vi "PID Robot Drive.vi"(8 "dt":dbl, 9 "Right RPS":dbl(slide) scale=-14.75..14.75, 10 "Left RPS":dbl(slide) scale=-14.75..14.75, 11 "Robot Mode Call Context":T1) -> (0 "Right Throttle":dbl, 3 "Left Throttle":dbl)   [LabVIEW 2016]
uses:
  <vilib>/Rock Robotics/WPI/DriverStation/WPI_DriverStationDerivedRobotMode.ctl
  <vilib>/Rock Robotics/Network Tables/NT Read Number.vi
  Robot Global Data.vi
  <vilib>/addons/control/pid/pid.llb/PID (DBL).vi
  <vilib>/addons/control/pid/NI_PID_pid.lvlib
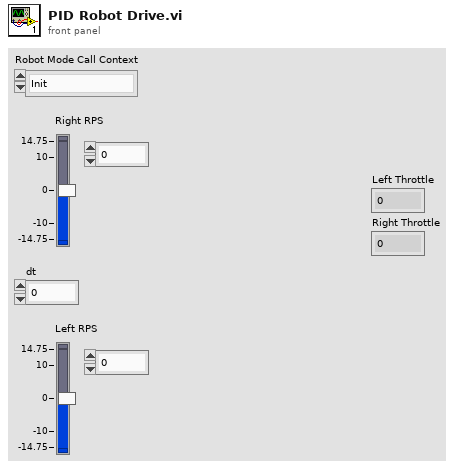
[diagram p1: front panel]
types:
  T1 = typedef "WPI_DriverStationDerivedRobotMode.ctl" = enum16{"Init", "Execute", "Stop"}
  T2 = cluster{"proportional gain (Kc)":dbl, "integral time (Ti, min)":dbl, "derivative time (Td, min)":dbl}
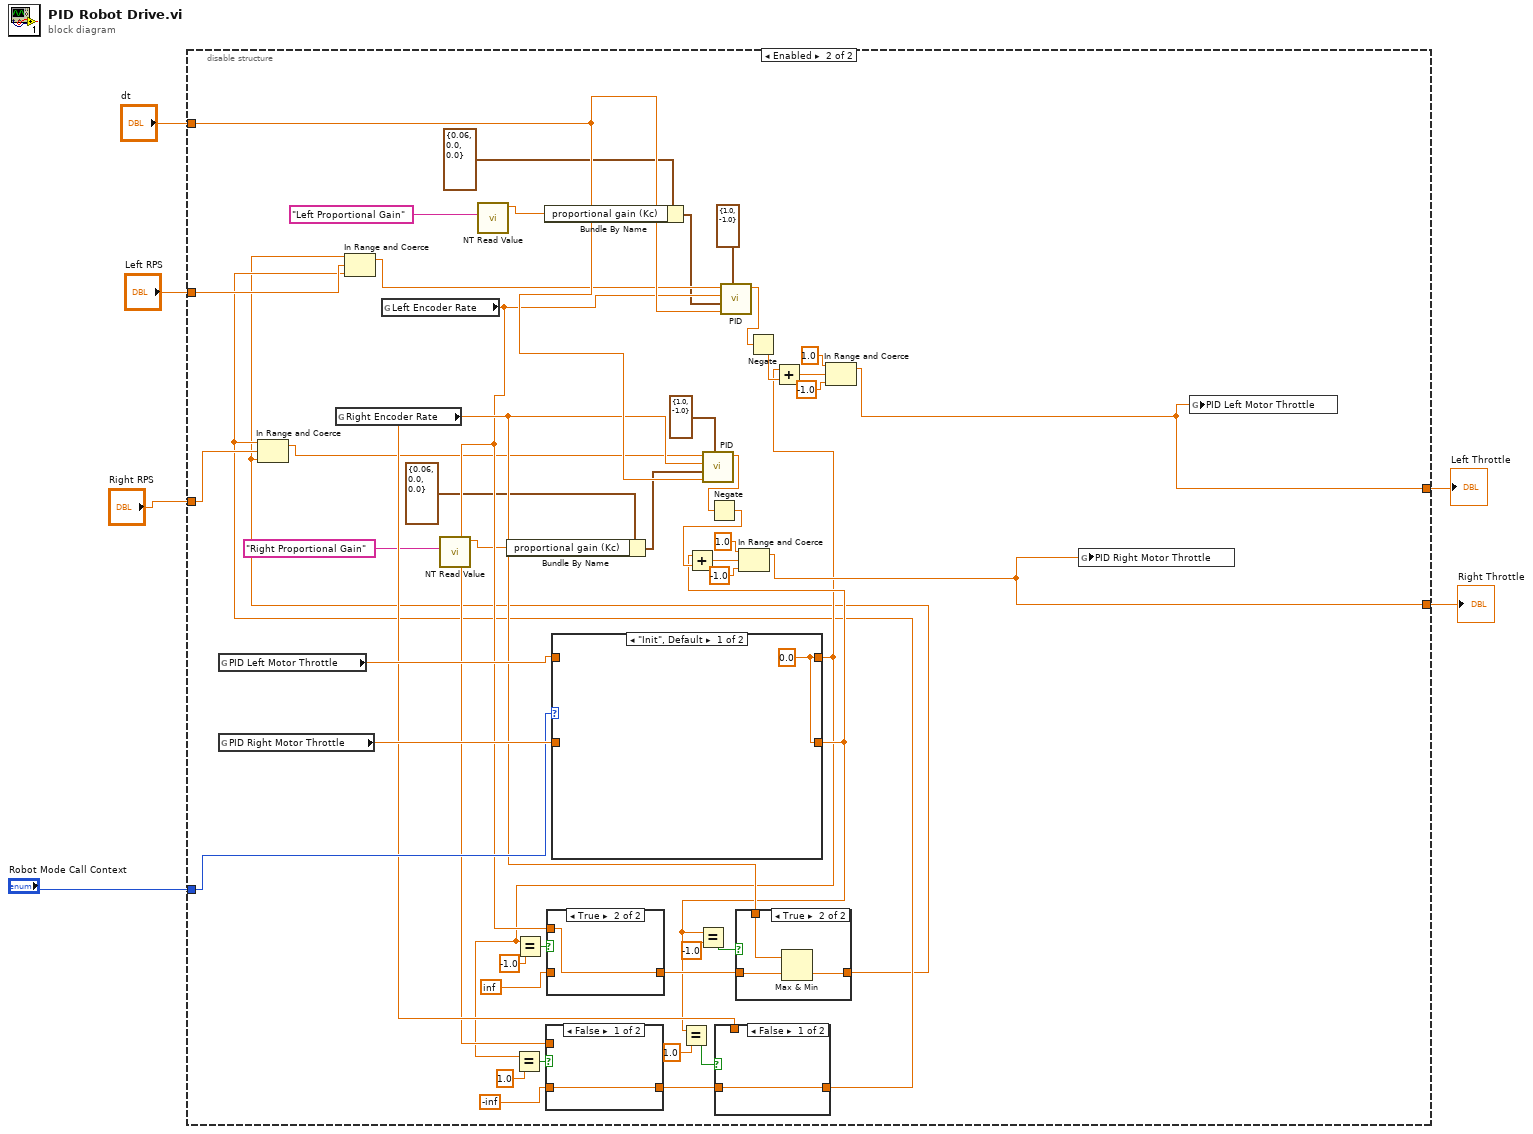
[diagram p0: block diagram]
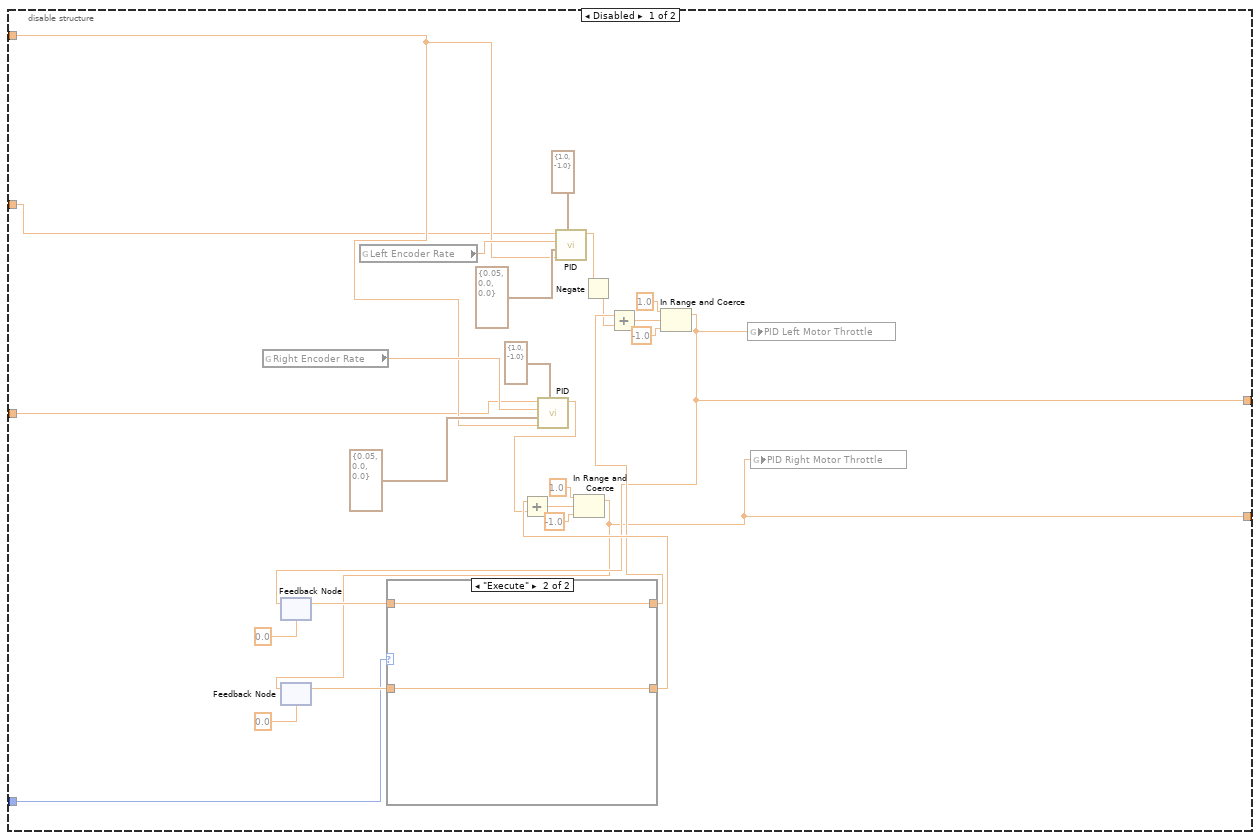
[diagram p2: hidden frame]
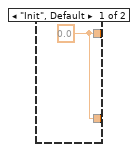
[diagram p3: hidden frame]
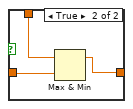
[diagram p4: hidden frame]
diagram:
  n1 = disable-structure shown="Enabled" {
    disable-tunnel: "dt" -> [w12 w74]
    disable-tunnel: "Right RPS" -> [w11 w49]
    disable-tunnel: "Left RPS" -> [w10 w51]
    disable-tunnel: [w9 w54] -> w3
    disable-tunnel: [w8 w53] -> w2
    disable-tunnel: "Robot Mode Call Context" -> [w7 w73]
    frame Disabled {
      n2 = global read "Robot Global Data.vi" "Right Encoder Rate"() -> (w27:dbl)
      n3 = feedback #1(0.0 ("TeleOp Elapsed Seconds")) -> (w29:dbl)
      n4 = feedback #2(0.0 ("TeleOp Elapsed Seconds")) -> (w32:dbl)
      n5 = global read "Robot Global Data.vi" "Left Encoder Rate"() -> (w14:dbl)
      n6 = case shown="\"Execute\"" w7 {
        tunnel: [w34 w36] -> w30
        tunnel: w29 -> [_ w36]
        tunnel: [w34 w35] -> w33
        tunnel: w32 -> [_ w35]
        frame "Init", Default {
          w34 = 0.0 ("TeleOp Elapsed Seconds")
        }
        frame "Execute" {
        }
      }
      n7 = call-poly <vilib>:"PID.vi"("output range"=cluster{"output high":dbl, "output low":dbl} {"output high"=1.0, "output low"=-1.0} ("Right output range"), "dt (s)"=w12, "PID gains"=T2 {"proportional gain (Kc)"=0.05, "integral time (Ti, min)"=0.0, "derivative time (Td, min)"=0.0} ("Right PID gains"), "process variable"=w27, "setpoint"=w11) -> ("output"=w25:dbl)  [unwired: 5 in, 1 out]
      n8 = Add(x=w33, y=w25) -> (x+y=w23:dbl)
      n9 = call-poly <vilib>:"PID.vi"("output range"=cluster{"output high":dbl, "output low":dbl} {"output high"=1.0, "output low"=-1.0} ("Left output range"), "dt (s)"=w12, "PID gains"=T2 {"proportional gain (Kc)"=0.05, "integral time (Ti, min)"=0.0, "derivative time (Td, min)"=0.0} ("Left PID gains"), "process variable"=w14, "setpoint"=w10) -> ("output"=w17:dbl)  [unwired: 5 in, 1 out]
      n10 = In Range and Coerce(upper limit=1.0, x=w23, lower limit=-1.0) -> (coerced(x)=w8:dbl)  [unwired: 1 out]
      n11 = feedback-in #2(w8) -> ()
      n12 = Negate(x=w17) -> (-x=w16:dbl)
      n13 = Add(x=w30, y=w16) -> (x+y=w18:dbl)
      n14 = In Range and Coerce(upper limit=1.0, x=w18, lower limit=-1.0) -> (coerced(x)=w9:dbl)  [unwired: 1 out]
      n15 = feedback-in #1(w9) -> ()
      n16 = global write "Robot Global Data.vi" "PID Left Motor Throttle"(w9) -> ()
      n17 = global write "Robot Global Data.vi" "PID Right Motor Throttle"(w8) -> ()
    }
    frame Enabled {
      n18 = global read "Robot Global Data.vi" "PID Left Motor Throttle"() -> (w76:dbl)
      n19 = global read "Robot Global Data.vi" "PID Right Motor Throttle"() -> (w75:dbl)
      n20 = global read "Robot Global Data.vi" "Right Encoder Rate"() -> (w56:dbl)
      n21 = global read "Robot Global Data.vi" "Left Encoder Rate"() -> (w55:dbl)
      n22 = call-poly <vilib>:"NT Read Value.vi"("Name"="Right Proportional Gain") -> ("Numeric"=w39:dbl)  [unwired: 9 in, 1 out]
      n23 = call-poly <vilib>:"NT Read Value.vi"("Name"="Left Proportional Gain") -> ("Numeric"=w42:dbl)  [unwired: 9 in, 1 out]
      n24 = Bundle By Name(cluster=T2 {"proportional gain (Kc)"=0.06, "integral time (Ti, min)"=0.0, "derivative time (Td, min)"=0.0} ("Left PID gains"), "proportional gain (Kc)"=w39) -> (w37:T2)
      n25 = Bundle By Name(cluster=T2 {"proportional gain (Kc)"=0.06, "integral time (Ti, min)"=0.0, "derivative time (Td, min)"=0.0} ("Left PID gains"), "proportional gain (Kc)"=w42) -> (w43:T2)
      n26 = case shown="\"Init\", Default" w73 {
        tunnel: [w97 w99] -> w47
        tunnel: w76 -> [_ w99]
        tunnel: [w97 w98] -> w52
        tunnel: w75 -> [_ w98]
        frame "Init", Default {
          w97 = 0.0 ("TeleOp Elapsed Seconds")
        }
        frame "Execute" {
        }
      }
      n27 = Equal?(x=w47, y=1.0) -> (x = y?=w62:bool)
      n28 = Equal?(x=w47, y=-1.0) -> (x = y?=w68:bool)
      n29 = case shown="False" w62 {
        tunnel: [w89 w90] -> w57
        tunnel: -inf -> [w89 _]
        tunnel: w55 -> [_ w90]
        frame False {
        }
        frame True {
        }
      }
      n30 = case shown="True" w68 {
        tunnel: [w95 w96] -> w63
        tunnel: inf -> [w95 _]
        tunnel: w55 -> [_ w96]
        frame False {
        }
        frame True {
        }
      }
      n31 = Equal?(x=w52, y=1.0) -> (x = y?=w58:bool)
      n32 = Equal?(x=w52, y=-1.0) -> (x = y?=w64:bool)
      n33 = case shown="False" w58 {
        tunnel: [w85 w86] -> w46
        tunnel: w57 -> [w85 w88]
        tunnel: w56 -> [_ w87]
        frame False {
        }
        frame True {
          n34 = Max & Min(x=w87, y=w88) -> (max(x,y)=w86:dbl)  [unwired: 1 out]
        }
      }
      n35 = case shown="True" w64 {
        tunnel: [w91 w92] -> w45
        tunnel: w63 -> [w91 w94]
        tunnel: w56 -> [_ w93]
        frame False {
        }
        frame True {
          n36 = Max & Min(x=w93, y=w94) -> (min(x,y)=w92:dbl)  [unwired: 1 out]
        }
      }
      n37 = In Range and Coerce(upper limit=w46, x=w49, lower limit=w45) -> (coerced(x)=w48:dbl)  [unwired: 1 out]
      n38 = In Range and Coerce(upper limit=w45, x=w51, lower limit=w46) -> (coerced(x)=w50:dbl)  [unwired: 1 out]
      n39 = call-poly <vilib>:"PID.vi"("output range"=cluster{"output high":dbl, "output low":dbl} {"output high"=1.0, "output low"=-1.0} ("Right output range"), "dt (s)"=w74, "PID gains"=w37, "process variable"=w56, "setpoint"=w48) -> ("output"=w70:dbl)  [unwired: 5 in, 1 out]
      n40 = Negate(x=w70) -> (-x=w69:dbl)
      n41 = Add(x=w52, y=w69) -> (x+y=w83:dbl)
      n42 = call-poly <vilib>:"PID.vi"("output range"=cluster{"output high":dbl, "output low":dbl} {"output high"=1.0, "output low"=-1.0} ("Left output range"), "dt (s)"=w74, "PID gains"=w43, "process variable"=w55, "setpoint"=w50) -> ("output"=w72:dbl)  [unwired: 5 in, 1 out]
      n43 = In Range and Coerce(upper limit=1.0, x=w83, lower limit=-1.0) -> (coerced(x)=w53:dbl)  [unwired: 1 out]
      n44 = Negate(x=w72) -> (-x=w71:dbl)
      n45 = Add(x=w47, y=w71) -> (x+y=w78:dbl)
      n46 = In Range and Coerce(upper limit=1.0, x=w78, lower limit=-1.0) -> (coerced(x)=w54:dbl)  [unwired: 1 out]
      n47 = global write "Robot Global Data.vi" "PID Right Motor Throttle"(w53) -> ()
      n48 = global write "Robot Global Data.vi" "PID Left Motor Throttle"(w54) -> ()
    }
  }
  "Left Throttle" <- w3
  "Right Throttle" <- w2
